vi "Configure Secured TCP Client.vi"(4 "Read Mode (Immediate)":T1(ring)=enum."Immediate", 6 "timeout ms":i32=5000, 7 "Hostname":string="localhost", 8 "error in (no error)":errorcluster, 9 "X.509 Certificate":path, 10 "remote port (443)":u16=443, 11 "address (localhost)":string="localhost") -> (0 "error out":errorcluster, 2 "Ready for SSL":bool, 3 "Secured TCP Connection":refnum<class "Connection.TCP-TLS.lvclass">)   [LabVIEW 2020, in "Connection.TCP-TLS.lvclass"]
uses:
  Connection.TCP-TLS.lvclass
  C:/Program Files (x86)/National Instruments/LabVIEW 2020/vi.lib/LabVIEW Open Source Project/MQTT TCP Connection/MQTT_TCP/Connection/TCPConnection.lvclass
  C:/Program Files (x86)/National Instruments/LabVIEW 2020/vi.lib/LabVIEW Open Source Project/MQTT Connection/MQTT_Connection/Connection/Connection.lvclass
  Connection.TCP-TLS.lvclass/Connection.TCP-TLS.ctl
  <vilib>/LabVIEW Open Source Project/MQTT TCP Connection/MQTT_TCP/Connection/TCPConnection.lvclass/TCPConnection.ctl
  <vilib>/LabVIEW Open Source Project/MQTT Connection/MQTT_Connection/Connection/Connection.lvclass/Connection.ctl
  <vilib>/LabVIEW Open Source Project/MQTT TCP Connection/MQTT_TCP/Connection/TCPConnection.lvclass
  <vilib>/LabVIEW Open Source Project/MQTT Connection/MQTT_Connection/Connection/Connection.lvclass
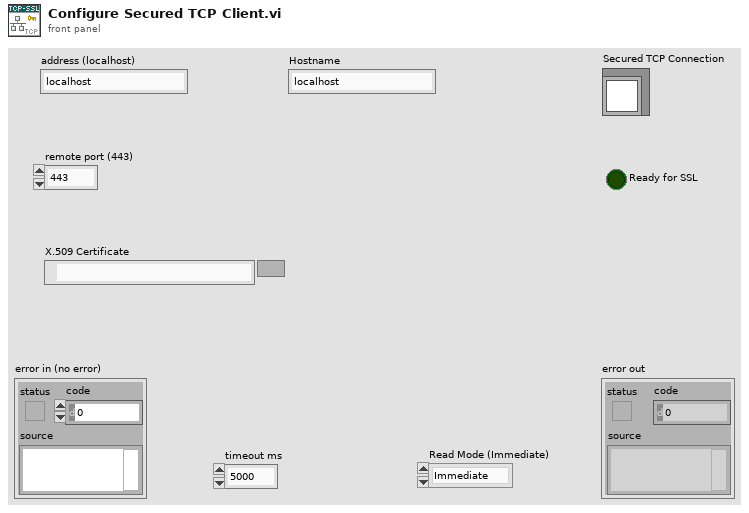
[diagram p1: front panel]
types:
  T1 = enum16{"Standard", "Buffered", "CRLF", "Immediate"}
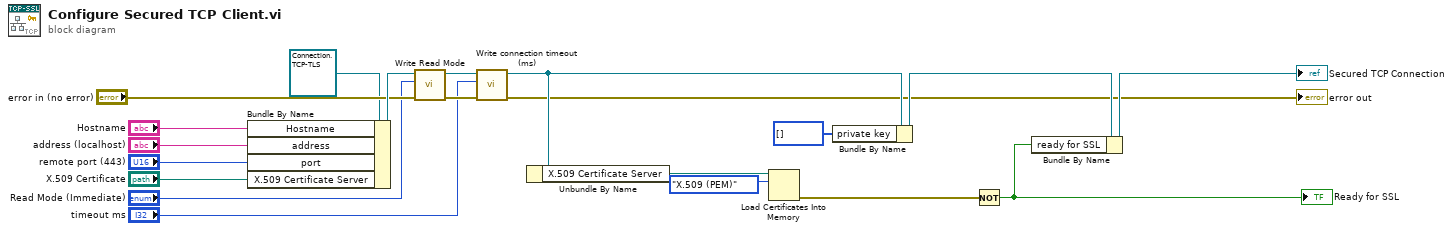
[diagram p0: block diagram]
diagram:
  n1 = Bundle By Name(cluster=refnum<class "Connection.TCP-TLS.lvclass"> refnum ("Connection.TCP-TLS in"), "Hostname"="Hostname", "address"="address (localhost)", "port"="remote port (443)", "X.509 Certificate Server"="X.509 Certificate") -> (w19:refnum<class "Connection.TCP-TLS.lvclass">)
  n2 = call <vilib>:"Write Read Mode.vi"("error in (no error)"="error in (no error)", "Read Mode"="Read Mode (Immediate)", "TCPConnection in"=w19) -> ("error out"=w18:errorcluster, "TCPConnection"=w20:refnum<class "Connection.TCP-TLS.lvclass">)  [unwired: 7 in]
  n3 = call <vilib>:"Write connection timeout (ms).vi"("error in (no error)"=w18, "connection timeout (ms)"="timeout ms", "Connection in"=w20) -> ("error out"=→"error out":errorcluster, "Connection out"=w15:refnum<class "Connection.TCP-TLS.lvclass">)  [unwired: 7 in]
  n4 = Unbundle By Name(w15) -> ("X.509 Certificate Server"=w16:path)
  n5 = Load Certificates Into Memory(10:enum32{"X.509 (PEM)"}."X.509 (PEM)" ("format"), 11:w16) -> (0:w3:errorcluster)  [unwired: 1 in, 1 out]
  n6 = Bundle By Name(cluster=w15, "private key"=u8[] []) -> (w14:refnum<class "Connection.TCP-TLS.lvclass">)
  n7 = Not(x=w3) -> (.not. x?=w10:bool)
  "Ready for SSL" <- w10
  n8 = Bundle By Name(cluster=w14, "ready for SSL"=w10) -> (→"Secured TCP Connection":refnum<class "Connection.TCP-TLS.lvclass">)
